vi "GetWaferData_Http.vi"(3 "error in (no error)":errorcluster, 5 "LotData in":refnum<class "LotData.lvclass">) -> (0 "error out":errorcluster, 1 "Array":T1[](array[typedef]) {"50mA Data"."Reverse" format="%#_3g"; "50mA Data"."Current,mA" format="%_6g"; "50mA Data"."Knee Current" format="%#_3g"; "50mA Data"."WL" format="%_6g"; "50mA Data"."Voltage" format="%_6g"; "50mA Data"."Power" format="%_5g"; "20mA Data"."Reverse" format="%#_3g"; "20mA Data"."Current,mA" format="%_6g"; "20mA Data"."Knee Current" format="%#_3g"; "20mA Data"."WL" format="%_6g"; "20mA Data"."Voltage" format="%_6g"; "20mA Data"."Power" format="%_5g"}, 2 "LotData out":refnum<class "LotData.lvclass">)   [LabVIEW 2012, in "LotData.lvclass"]
uses:
  LotData.lvclass
  Controls/TestData.ctl
  Controls/Measurement.ctl
  Controls/PadArea.ctl
  LotData.lvclass/LotData.ctl
  <vilib>/LVH/i3 JSON/JSON Parsing/Get Object Parameter Files/Get Object Parameter - JSON Tree.vi
  <vilib>/LVH/i3 JSON/JSON Parsing/Get Object Parameter Files/Get Object Parameter - String.vi
  <vilib>/LVH/i3 JSON/JSON Parsing/Get Object Parameter Files/Get Object Parameter - Numeric.vi
  <vilib>/LVH/i3 JSON/i3-json.lvlib
  <vilib>/httpClient/LabVIEWHTTPClient.lvlib
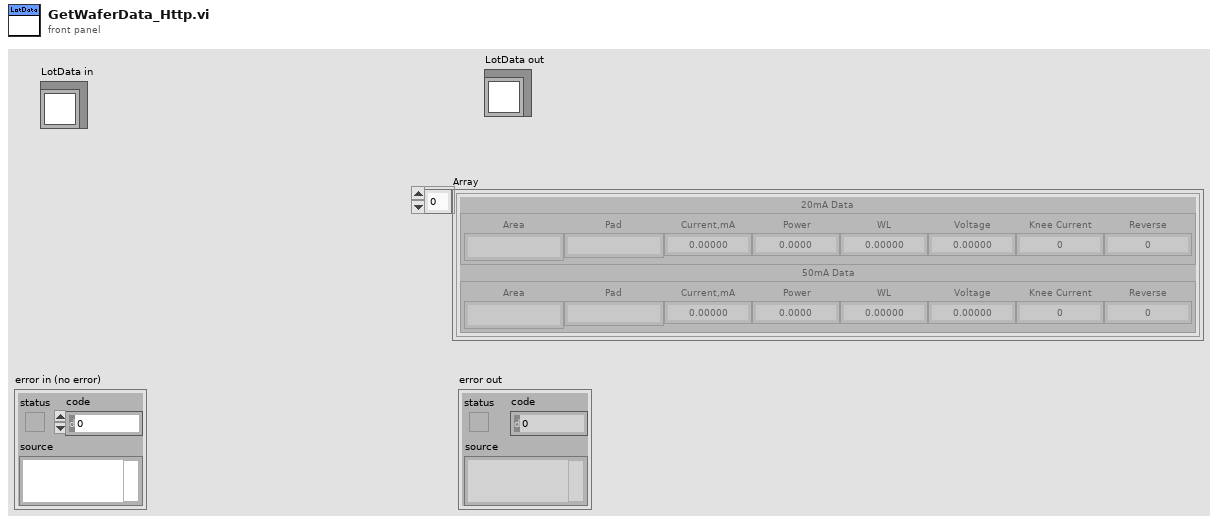
[diagram p1: front panel]
types:
  T1 = typedef "TestData.ctl" = cluster{"20mA Data":T2, "50mA Data ":T2}
  T2 = typedef "Measurement.ctl" = cluster{"Area":string, "Pad":string, "Current,mA":dbl, "Power":dbl, "WL":dbl, "Voltage":dbl, "Knee Current":dbl, "Reverse":dbl}
  T3 = typedef "PadArea.ctl" = enum16{"A", "B", "C", "D", "L", "R", "T", "G"}
  T4 = typedef "LabVIEWHTTPClient.lvlib/ClientHandle.ctl" = refnum<k1>
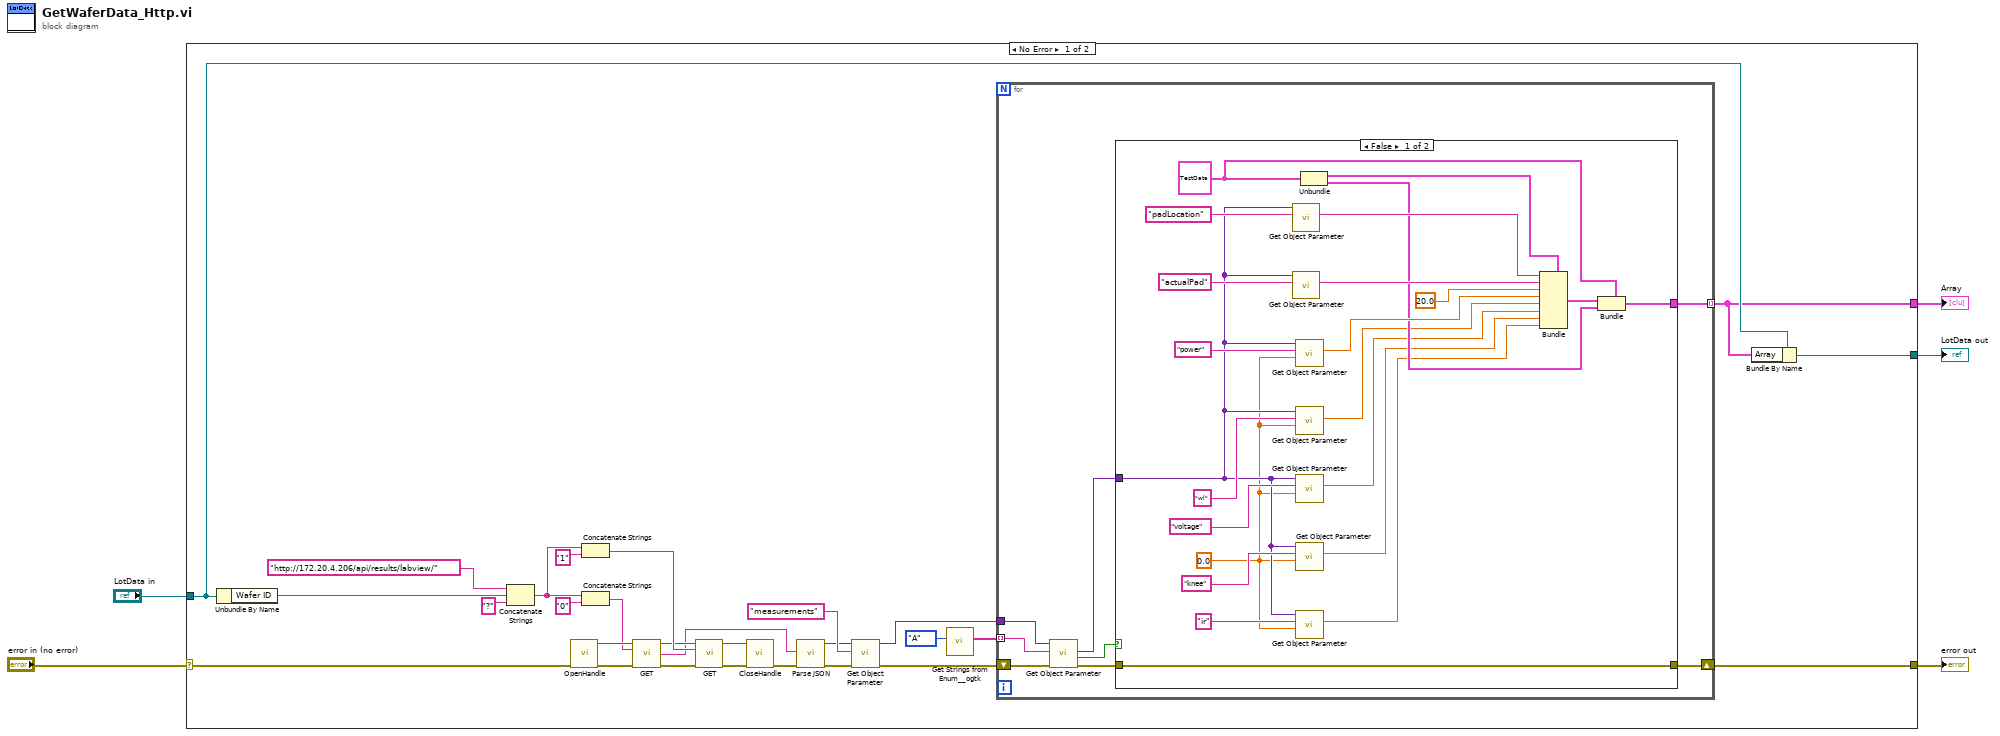
[diagram p0: block diagram]
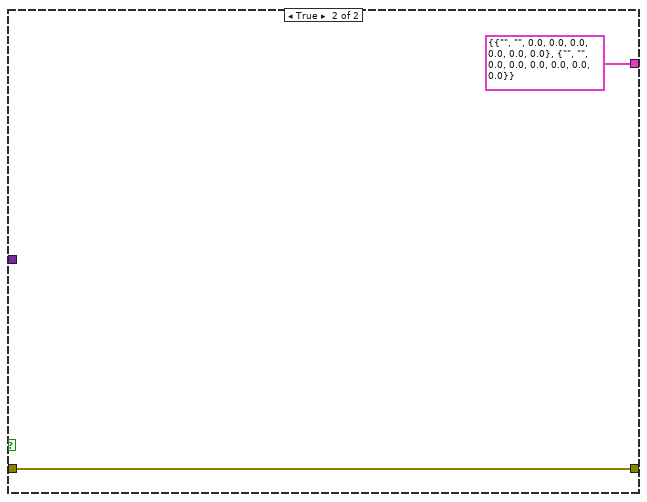
[diagram p2: hidden frame]
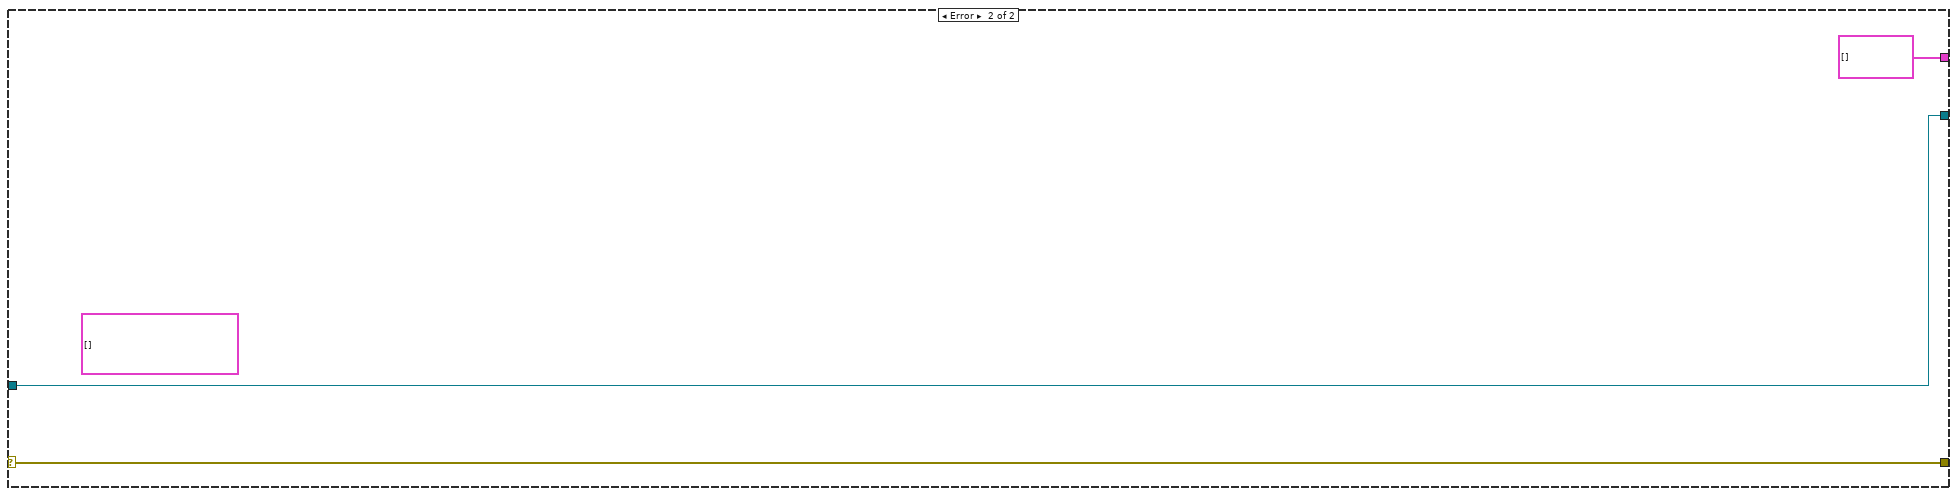
[diagram p3: hidden frame]
diagram:
  n1 = case shown="No Error" "error in (no error)" {
    selector: "error in (no error)" -> [w32 w69]
    tunnel: [w9 w69] -> w3
    tunnel: [w11 w68] -> w2
    tunnel: "LotData in" -> [w10 w68]
    tunnel: [w8 T1[] []] -> w1
    frame No Error {
      n2 = Unbundle By Name(w10) -> ("Wafer ID"=w33:string)
      n3 = Concatenate Strings("http://172.20.4.206/api/results/labview/" ("url"), w33, "?" ("string")) -> (w27:string)
      n4 = call <vilib>:"OpenHandle.vi"("error in (no error)"=w32) -> ("client handle out"=w31:T4, "error out"=w30:errorcluster)  [unwired: 13 in]
      n5 = Concatenate Strings(w27, "1" ("string")) -> (w22:string)
      n6 = Concatenate Strings(w27, "0" ("string")) -> (w23:string)
      n7 = call <vilib>:"GET.vi"("client handle"=w31, "url"=w23, "error in (no error)"=w30) -> ("client handle out"=w21:T4, "body"=w19:string, "error out"=w20:errorcluster)  [unwired: 9 in, 1 out]
      n8 = call <vilib>:"GET.vi"("client handle"=w21, "url"=w22, "error in (no error)"=w20) -> ("client handle out"=w17:T4, "error out"=w18:errorcluster)  [unwired: 9 in, 2 out]
      n9 = call <vilib>:"CloseHandle.vi"("client handle"=w17, "error in (no error)"=w18) -> ("error out"=w16:errorcluster)  [unwired: 13 in]
      n10 = call <vilib>:"Parse JSON.vi"("error in (no error)"=w16, "JSON String"=w19) -> ("error out"=w6:errorcluster, "JSON Tree"=w7:variant)  [unwired: 6 in, 2 out]
      n11 = call-poly <vilib>:"Get Object Parameter.vi"("error in (no error)"=w6, "Parameter Name"="measurements", "JSON Tree In (JSON Object)"=w7) -> ("error out"=w12:errorcluster, "JSON Tree Out Passthrough"=w13:variant)  [unwired: 5 in, 2 out]
      n12 = call <userlib>:"Get Strings from Enum__ogtk.vi"("Enum"=PadArea."A" ("PadArea")) -> ("Enum Strings"=w14:string[])  [unwired: 7 in, 3 out]
      n13 = for {
        tunnel: w14 -> [w40] mode=indexing
        tunnel: w13 -> [w39]
        shift-right: [w35] -> w9
        shift-left: w12 -> [w38]
        tunnel: [w34] -> w8 mode=indexing
        n14 = call-poly <vilib>:"Get Object Parameter.vi"("error in (no error)"=w38, "Parameter Name"=w40, "JSON Tree In (JSON Object)"=w39) -> ("error out"=w36:errorcluster, "is JSON Null?"=w37:bool, "JSON Value (JSON Tree)"=w41:variant)  [unwired: 5 in, 1 out]
        n15 = case shown="False" w37 {
          tunnel: w41 -> [w57 _]
          tunnel: [w53 w66] -> w35
          tunnel: w36 -> [w53 w66]
          tunnel: [w48 T1 {"20mA Data"={"Area"="", "Pad"="", "Current,mA"=0.0, "Power"=0.0, "WL"=0.0, "Voltage"=0.0, "Knee Current"=0.0, "Reverse"=0.0}, "50mA Data "={"Area"="", "Pad"="", "Current,mA"=0.0, "Power"=0.0, "WL"=0.0, "Voltage"=0.0, "Knee Current"=0.0, "Reverse"=0.0}} ("TestData")] -> w34
          frame False {
            w42 = 0.0 ("Default Value if JSON Null")
            w51 = T1 {"20mA Data"={"Area"="", "Pad"="", "Current,mA"=0.0, "Power"=0.0, "WL"=0.0, "Voltage"=0.0, "Knee Current"=0.0, "Reverse"=0.0}, "50mA Data "={"Area"="", "Pad"="", "Current,mA"=0.0, "Power"=0.0, "WL"=0.0, "Voltage"=0.0, "Knee Current"=0.0, "Reverse"=0.0}} ("TestData")
            n16 = call-poly <vilib>:"Get Object Parameter.vi"("Parameter Name"="padLocation", "JSON Tree In (JSON Object)"=w57) -> ("String Value"=w56:string)  [unwired: 6 in, 3 out]
            n17 = call-poly <vilib>:"Get Object Parameter.vi"("Parameter Name"="actualPad", "JSON Tree In (JSON Object)"=w57) -> ("String Value"=w55:string)  [unwired: 6 in, 3 out]
            n18 = call-poly <vilib>:"Get Object Parameter.vi"("Default Value if JSON Null"=w42, "Parameter Name"="power", "JSON Tree In (JSON Object)"=w57) -> ("Double Value"=w54:dbl)  [unwired: 5 in, 3 out]
            n19 = call-poly <vilib>:"Get Object Parameter.vi"("Default Value if JSON Null"=w42, "Parameter Name"="wl", "JSON Tree In (JSON Object)"=w57) -> ("Double Value"=w46:dbl)  [unwired: 5 in, 3 out]
            n20 = call-poly <vilib>:"Get Object Parameter.vi"("Default Value if JSON Null"=w42, "Parameter Name"="voltage", "JSON Tree In (JSON Object)"=w57) -> ("Double Value"=w45:dbl)  [unwired: 5 in, 3 out]
            n21 = call-poly <vilib>:"Get Object Parameter.vi"("Default Value if JSON Null"=w42, "Parameter Name"="knee", "JSON Tree In (JSON Object)"=w57) -> ("Double Value"=w44:dbl)  [unwired: 5 in, 3 out]
            n22 = call-poly <vilib>:"Get Object Parameter.vi"("Default Value if JSON Null"=w42, "Parameter Name"="ir", "JSON Tree In (JSON Object)"=w57) -> ("Double Value"=w43:dbl)  [unwired: 5 in, 3 out]
            n23 = Unbundle(w51) -> ("20mA Data"=w52:T2, "50mA Data"=w49:T2)
            n24 = Bundle(cluster=w52, "Area"=w56, "Pad"=w55, "Current,mA"=20.0, "Power"=w54, "WL"=w46, "Voltage"=w45, "Knee Current"=w44, "Reverse"=w43) -> (w50:T2)
            n25 = Bundle(cluster=w51, "20mA Data"=w50, "50mA Data"=w49) -> (w48:T1)
          }
          frame True {
          }
        }
      }
      n26 = Bundle By Name(cluster=w10, "Array"=w8) -> (w11:refnum<class "LotData.lvclass">)
    }
    frame Error {
      (unwired) T1[] []
    }
  }
  "error out" <- w3
  "LotData out" <- w2
  "Array" <- w1
